vi "Perform Gain and Offset Measurements.vi"(7 "Measurement Context":refnum<class "Measure Call Context.lvclass">, 8 "error in":errorcluster, 10 "measurement configuration":T4={"Input channel"=0, "Full scale range"=10.0, "Analog source resource name"="", "Analog source sample rate"=800000.0, "Ramp samples"=-1, "Ramp start"=1000.0, "Ramp stop"=-1.0, "Digital capture resource name"="", "Digital capture sample rate"=800000.0, "Digital capture samples"=800000, "DMM resource name"="", "DMM range"=800000.0, "DMM resolution"=800000.0}, 11 "device sessions":T2) -> (0 "error out":errorcluster, 2 "measurement results":T3)   [LabVIEW 2021, in "adc_gainAndOffsetMeasurement.lvlib"]
uses:
  adc_gainAndOffsetMeasurement.lvlib
  Measurement Configuration.ctl
  Measurement Results.ctl
  <vilib>/MeasurementLink/MeasurementLink Measurement Server/Measure Call Context/Measure Call Context.lvclass
  <vilib>/gRPC/LabVIEW gRPC Library/Shared/grpcId.ctl
  <vilib>/Analysis/1siggen.llb/Ramp Pattern by Samples.vi
  <vilib>/DAQmx/write.llb/DAQmx Write (Analog 1D DBL 1Chan NSamp).vi
  <vilib>/Analysis/baseanly.llb/Mean (DBL).vi
  <vilib>/MeasurementLink/MeasurementLink Measurement Server/Measure Call Context/Accessor/Is Canceled.vi
  <vilib>/DAQmx/miscellaneous.llb/DAQmx Fill In Error Info.vi
  <vilib>/Analysis/NI_AALBase.lvlib
  <vilib>/Analysis/NI_AALPro.lvlib
  shared/digitalInterface/client/dcvmDPI_AD7606B_clientImpl/dcvmDPI_AD7606B_clientImpl.lvlib
  <vilib>/gRPC/LabVIEW gRPC Library/grpc-lvsupport-release.lvlib
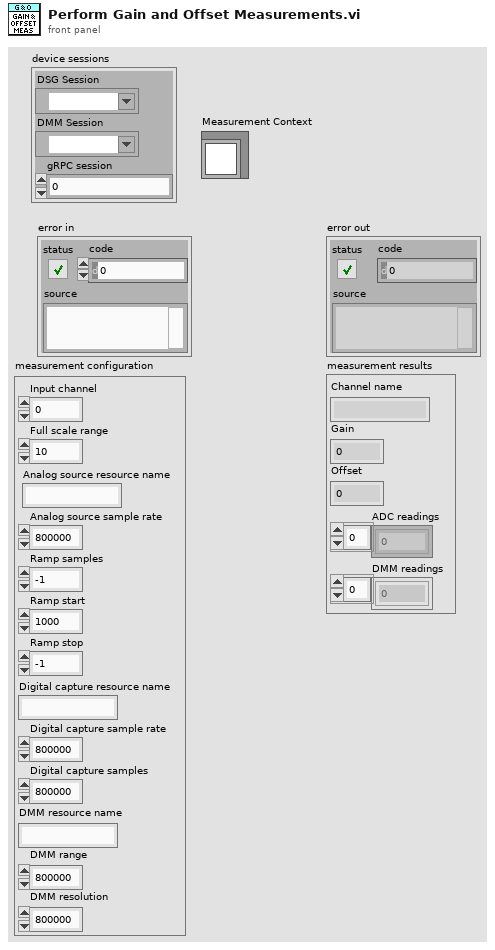
[diagram p1: front panel]
types:
  T1 = typedef "grpc-lvsupport-release.lvlib/grpcId.ctl" = u64
  T2 = cluster{"DSG Session":refnum<k21>, "DMM Session":refnum<k15>, "gRPC session":T1}
  T3 = typedef "adc_gainAndOffsetMeasurement.lvlib/Measurement Results.ctl" = cluster{"Channel name":string, "Gain":dbl, "Offset":dbl, "ADC readings":dbl[], "DMM readings":dbl[]}
  T4 = typedef "adc_gainAndOffsetMeasurement.lvlib/Measurement Configuration.ctl" = cluster{"Input channel":i32, "Full scale range":dbl, "Analog source resource name":string, "Analog source sample rate":dbl, "Ramp samples":i32, "Ramp start":dbl, "Ramp stop":dbl, "Digital capture resource name":string, "Digital capture sample rate":dbl, "Digital capture samples":u32, "DMM resource name":string, "DMM range":dbl, "DMM resolution":dbl}
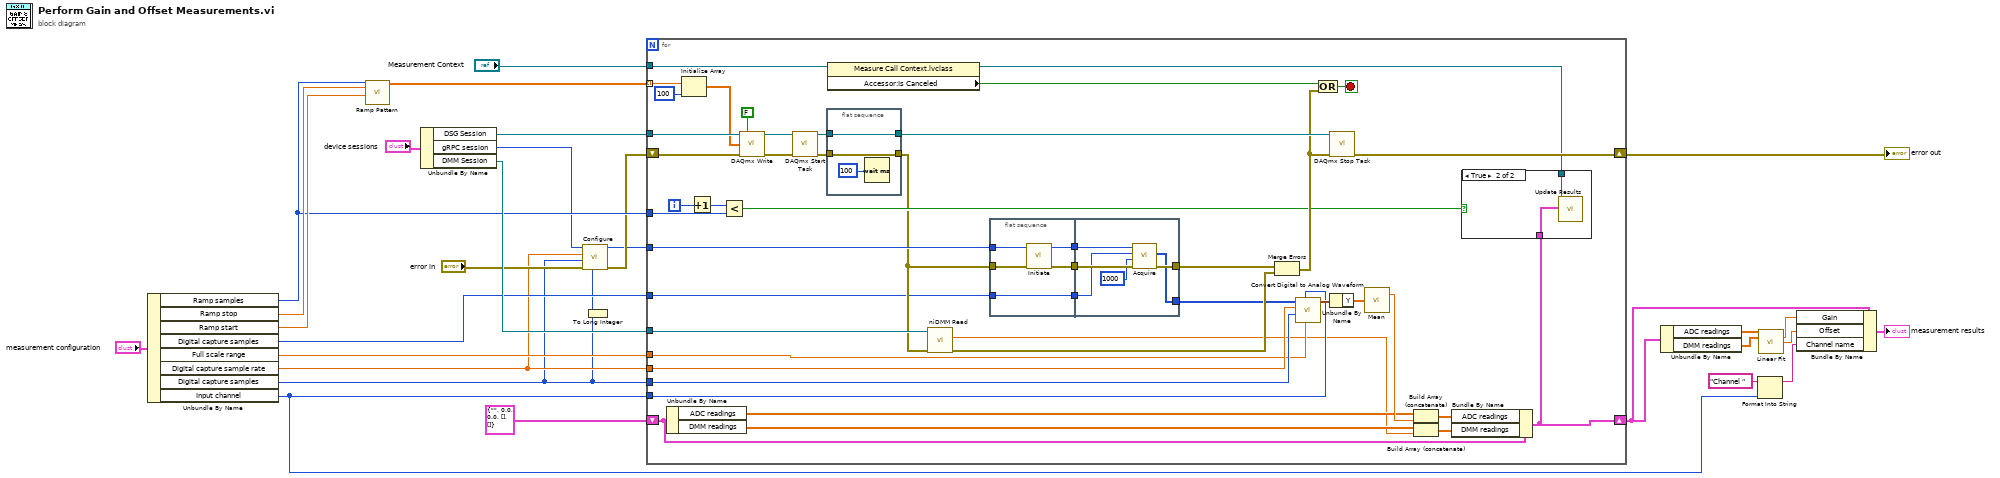
[diagram p0: block diagram]
diagram:
  n1 = Unbundle By Name("measurement configuration") -> ("Ramp samples"=w9:i32, "Ramp stop"=w24:dbl, "Ramp start"=w23:dbl, "Digital capture samples"=w22:u32, "Full scale range"=w16:dbl, "Digital capture sample rate"=w2:dbl, "Digital capture samples"=w1:u32, "Input channel"=w14:i32)
  n2 = call-poly <vilib>:"Ramp Pattern.vi"("start"=w23, "end"=w24, "samples"=w9) -> ("Ramp Pattern"=w29:dbl[])  [unwired: 7 in, 1 out]
  n3 = Unbundle By Name("device sessions") -> ("DSG Session"=w28:refnum<k21>, "gRPC session"=w7:T1, "DMM Session"=w27:refnum<k15>)
  n4 = To Long Integer(number=w1) -> (32bit integer=w6:i32)
  n5 = call "Configure.vi"("Input channel"=w6, "error in"="error in", "Digital capture samples"=w1, "Digital capture sample rate"=w2, "gRPC session in"=w7) -> ("error out"=w4:errorcluster, "gRPC session out"=w3:T1)  [unwired: 5 in]
  n6 = for {
    tunnel: w29 -> [w74] mode=indexing
    tunnel: w22 -> [w33]
    tunnel: w2 -> [w64]
    tunnel: w1 -> [w63]
    shift-right: [w58] -> w25
    shift-left: w4 -> [w57]
    tunnel: w16 -> [w55]
    tunnel: "Measurement Context" -> [w54]
    tunnel: w28 -> [w72]
    tunnel: w27 -> [w65]
    tunnel: w14 -> [w56]
    shift-right: [w39] -> w12
    shift-left: T3 {"Channel name"="", "Gain"=0.0, "Offset"=0.0, "ADC readings"=[], "DMM readings"=[]} ("Measurement Results") -> [w46]
    tunnel: w9 -> [w41]
    tunnel: w3 -> [w37]
    i -> [w43]
    stop <- w51 stop-if-true
    n7 = Unbundle By Name(w46) -> ("ADC readings"=w49:dbl[], "DMM readings"=w48:dbl[])
    n8 = Initialize Array(w74, 100 ("dimension size")) -> (w66:dbl[])
    n9 = Increment(x=w43) -> (x+1=w42:i32)
    n10 = Less?(x=w42, y=w41) -> (x < y?=w38:bool)
    n11 = call-poly <vilib>:"DAQmx Write.vi"("task/channels in"=w72, "auto start"=FALSE, "data"=w66, "error in"=w57) -> ("task out"=w70:refnum<k21>, "error out"=w69:errorcluster)  [unwired: 9 in, 1 out]
    n12 = call <vilib>:"DAQmx Start Task.vi"("task/channels in"=w70, "error in"=w69) -> ("task out"=w67:refnum<k21>, "error out"=w68:errorcluster)  [unwired: 12 in]
    n13 = flat-sequence {
      tunnel: w68 -> [w88]
      tunnel: w67 -> [w89]
      tunnel: [w89] -> w60
      tunnel: [w88] -> w36
      frame #0 {
        n14 = Wait (ms)(milliseconds to wait=u32 100) -> ()  [unwired: 1 out]
      }
    }
    n15 = property class="Measure Call Context.lvclass"(reference=w54) -> (reference out=w40:refnum<class "Measure Call Context.lvclass">, "Accessor:Is Canceled"=w52:bool)  [unwired: 1 in, 1 out]
    n16 = call <instrlib>:"niDMM Read.vi"("error in (no error)"=w36, "instrument handle"=w65) -> ("error out"=w61:errorcluster, "Measurement"=w47:dbl)  [unwired: 7 in, 1 out]
    n17 = flat-sequence {
      tunnel: w37 -> [w79]
      tunnel: w36 -> [w78]
      tunnel: [w77] -> w35
      tunnel: [w76] -> w34
      tunnel: w33 -> [w75]
      tunnel: [w75] -> w32
      tunnel: w35 -> [w85]
      tunnel: w34 -> [w84]
      tunnel: w32 -> [w83]
      tunnel: [w81] -> w31
      tunnel: [w80] -> w30
      frame #0 {
        n18 = call "Initiate.vi"("error in"=w78, "gRPC session in"=w79) -> ("error out"=w76:errorcluster, "gRPC session out"=w77:T1)  [unwired: 8 in]
      }
      frame #1 {
        n19 = call "Acquire.vi"("error in"=w84, "Timeout (ms)"=1000, "Digital capture samples"=w83, "gRPC session in"=w85) -> ("error out"=w81:errorcluster, "Digital waveform"=w80:u32[])  [unwired: 5 in, 1 out]
      }
    }
    n20 = Merge Errors(w31, w61) -> (w53:errorcluster)
    n21 = call "Convert Digital to Analog Waveform.vi"("full scale range"=w55, "channel index"=w56, "Number of samples"=w63, "Sample rate"=w64, "Digital waveform in"=w30) -> ("Waveform"=w62:waveform(dbl))  [unwired: 4 in, 2 out]
    n22 = Compound Arithmetic op=OR(w52, w53) -> (w51:bool)
    n23 = call <vilib>:"DAQmx Stop Task.vi"("task/channels in"=w60, "error in"=w53) -> ("error out"=w58:errorcluster)  [unwired: 12 in, 1 out]
    n24 = Unbundle By Name(w62) -> ("Y"=w59:dbl[])
    n25 = call-poly <vilib>:"Mean.vi"("X"=w59) -> ("mean"=w50:dbl)  [unwired: 1 out]
    n26 = Build Array (concatenate)(w49, w50) -> (w45:dbl[])
    n27 = Build Array (concatenate)(w48, w47) -> (w44:dbl[])
    n28 = Bundle By Name(cluster=w46, "ADC readings"=w45, "DMM readings"=w44) -> (w39:T3)
    n29 = case shown="True" w38 {
      tunnel: w40 -> [_ w87]
      tunnel: w39 -> [_ w86]
      frame False {
      }
      frame True {
        n30 = call <vilib>:"Update Results.vi"("measurement results"=w86, "measure call context in"=w87) -> ()  [unwired: 8 in, 2 out]
      }
    }
  }
  "error out" <- w25
  n31 = Unbundle By Name(w12) -> ("ADC readings"=w11:dbl[], "DMM readings"=w10:dbl[])
  n32 = Format Into String(initial string="Channel ", w14) -> (resulting string=w18:string)  [unwired: 2 in, 1 out]
  n33 = call <vilib>:"Linear Fit.vi"("Y"=w11, "X"=w10) -> ("slope"=w20:dbl, "intercept"=w21:dbl)  [unwired: 9 in, 3 out]
  n34 = Bundle By Name(cluster=w12, "Gain"=w20, "Offset"=w21, "Channel name"=w18) -> (→"measurement results":T3)
